vi "ValidateMove.vi"(8 "error in (no error)":errorcluster, 10 "targetMove":dbl, 11 "KST101 in":refnum<class "KST101.lvclass">) -> (0 "error out":errorcluster, 2 "validMove?":bool, 3 "KST101 out":refnum<class "KST101.lvclass">)   [LabVIEW 2016, in "Stepper Motor Controller.lvlib" / "KST101.lvclass"]
uses:
  KST101.lvclass
  KST101.lvclass/KST101.ctl
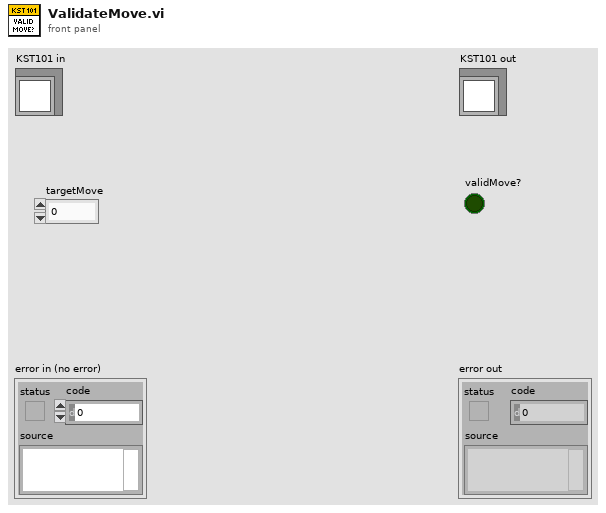
[diagram p1: front panel]
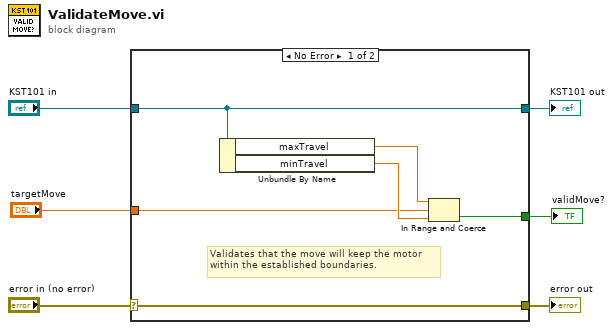
[diagram p0: block diagram]
diagram:
  n1 = case shown="No Error" "error in (no error)" {
    selector: "error in (no error)" -> [w12 w14]
    tunnel: [w12 w14] -> w5
    tunnel: [w9 w13] -> w3
    tunnel: "KST101 in" -> [w9 w13]
    tunnel: "targetMove" -> [w8 _]
    tunnel: [w7 _] -> w1
    frame No Error {
      # "Validates that the move will keep the motor\nwithin the established boundaries."
      n2 = Unbundle By Name(w9) -> ("maxTravel"=w11:dbl, "minTravel"=w10:dbl)
      n3 = In Range and Coerce(upper limit=w11, x=w8, lower limit=w10) -> (In Range?=w7:bool)  [unwired: 1 out]
    }
    frame Error {
    }
  }
  "error out" <- w5
  "KST101 out" <- w3
  "validMove?" <- w1
